vi "Chebeval2.vi"(10 "Cheby weights":dbl[](array[numeric]), 11 "x":dbl[](array[numeric])) -> (3 "y":dbl[](array[numeric]))   [LabVIEW 2019]
panel:
  out "Array":dbl[][](array[numeric])
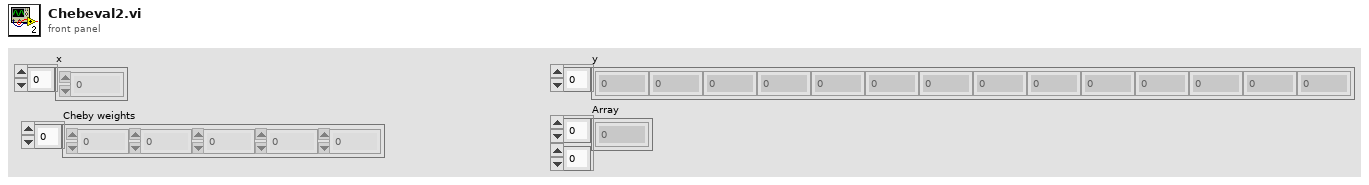
[diagram p1: front panel]
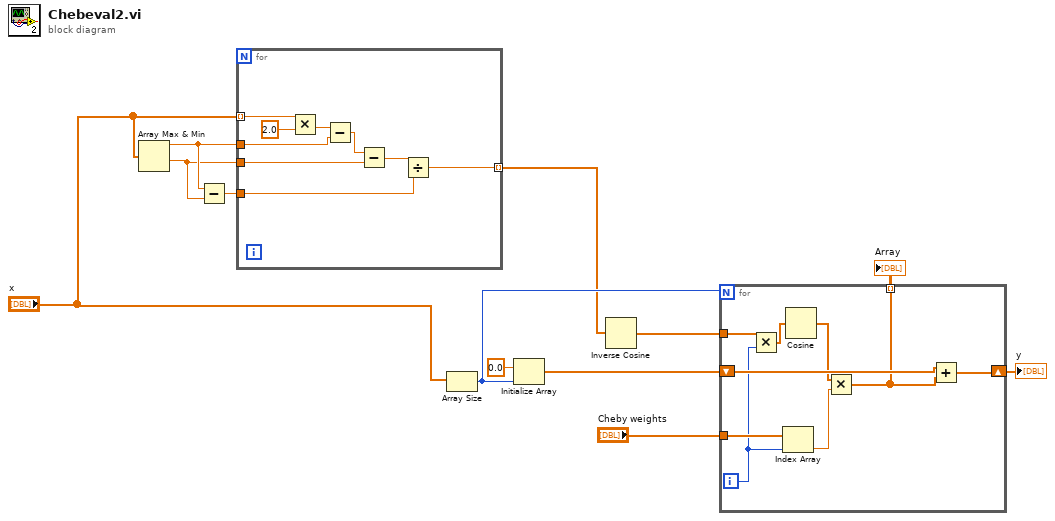
[diagram p0: block diagram]
diagram:
  n1 = Array Max & Min(array="x") -> (max value=w10:dbl, min value=w9:dbl)  [unwired: 2 out]
  n2 = Subtract(x=w10, y=w9) -> (x-y=w8:dbl)
  n3 = for {
    tunnel: "x" -> [w21] mode=indexing
    tunnel: w10 -> [w18]
    tunnel: w9 -> [w16]
    tunnel: w8 -> [w14]
    tunnel: [w13] -> w3 mode=indexing
    n4 = Multiply(x=w21, y=2.0) -> (x*y=w19:dbl)
    n5 = Subtract(x=w19, y=w18) -> (x-y=w17:dbl)
    n6 = Subtract(x=w17, y=w16) -> (x-y=w15:dbl)
    n7 = Divide(x=w15, y=w14) -> (x/y=w13:dbl)
  }
  n8 = Array Size(array="x") -> (size(s)=w11:i32)
  n9 = Initialize Array(0.0 ("element"), w11) -> (w7:dbl[])
  n10 = Inverse Cosine(1:w3) -> (0:w5:dbl[])
  n11 = for {
    N: w11 -> [_]
    shift-right: [w26] -> w2
    shift-left: w7 -> [w27]
    tunnel: w5 -> [w30]
    tunnel: "Cheby weights" -> [w29]
    tunnel: [w25] -> w1 mode=indexing
    i -> [w22]
    n12 = Multiply(x=w30, y=w22) -> (x*y=w24:dbl[])
    n13 = Index Array(array=w29, index=w22) -> (element=w28:dbl)
    n14 = Cosine(x=w24) -> (cos(x)=w23:dbl[])
    n15 = Multiply(x=w23, y=w28) -> (x*y=w25:dbl[])
    n16 = Add(x=w27, y=w25) -> (x+y=w26:dbl[])
  }
  "y" <- w2
  "Array" <- w1
